vi "SPI MPU9250.vi"() -> ()   [LabVIEW 2020, in "CTI-Scratchpad.lvlib"]
uses:
  CTI-Scratchpad.lvlib
  CTI/SPI Config.ctl
  CTI/SPI Mode.ctl
  CTI/SPI Pins.ctl
  CTI/GPIO Number.ctl
  CTI/SPI Number.ctl
  CTI/GPIO Direction.ctl
  CTI/Session/Session.lvclass
  6879a345-385a-4bff-b9a2-dde094eab613.vi
  CTI/SPI/SPI.lvclass
  CTI/VisaComms/VisaComms.lvclass
  CTI/SPI CS/SPI CS.lvclass
  CTI/CTI.lvlib
panel:
  out "ID":string
  out "Chart":T1(graph)
  in  "stop":bool
  out "error out":errorcluster={"status"=FALSE, "code"=1073676294, "source"="VISA Read in CTI-Visa.lvlib:Read Response.vi->CTI-Visa.lvlib:Read SPI.vi->CTI-Visa-DeviceLib.lvlib:SPI Read Register.vi->CTI-Visa-Scratchpad.lvlib:SPI MPU9250.vi"}
  in  "CS GPIO":T2=5
  in  "Baud":u32=500000 format="%.0p"
  in  "SPI #":T3
  in  "SPI Config":T4={"Mode"=0, "Data Bits"=8, "Pins"={"TX GPIO"=7, "RX GPIO"=4, "SCK GPIO"=6}}
  in  "Port":refnum<visa-resource-name>="COM4"
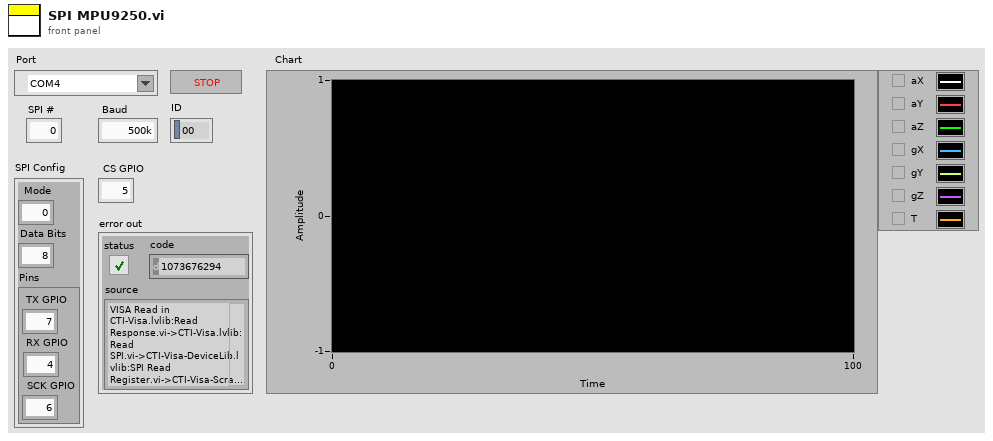
[diagram p1: front panel]
types:
  T1 = cluster{"X":u16, "Y":u16, "Z":u16, "X":u16, "Y":u16, "Z":u16, "T":u16}
  T2 = typedef "CTI.lvlib/GPIO Number.ctl" = i8
  T3 = typedef "CTI.lvlib/SPI Number.ctl" = i8
  T4 = typedef "CTI.lvlib/SPI Config.ctl" = cluster{"Mode":T5, "Data Bits":i8, "Pins":T6}
  T5 = typedef "CTI.lvlib/SPI Mode.ctl" = i8
  T6 = typedef "CTI.lvlib/SPI Pins.ctl" = cluster{"TX GPIO":T2, "RX GPIO":T2, "SCK GPIO":T2}
  T7 = typedef "CTI.lvlib/GPIO Direction.ctl" = enum16{"In", "Out"}
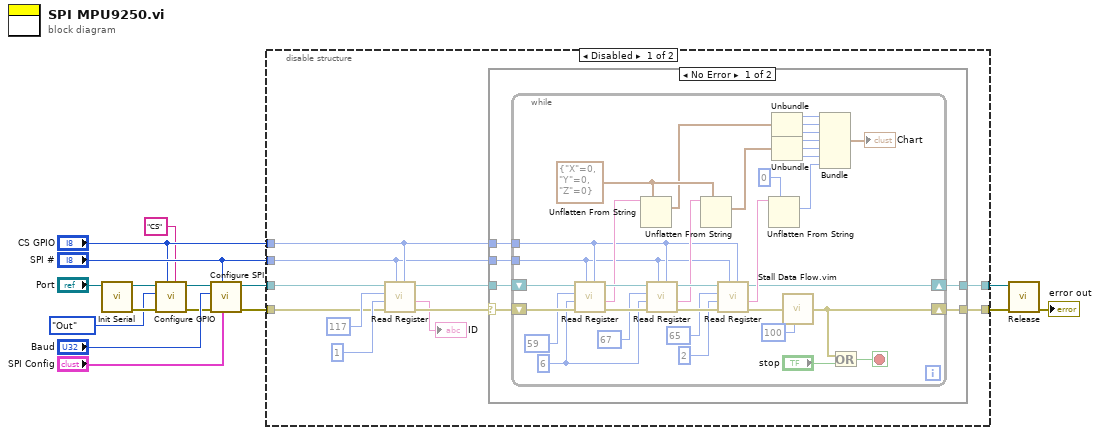
[diagram p0: block diagram]
diagram:
  n1 = call "Init Serial.vi"("VISA resource name in"="Port") -> ("error out"=w8:errorcluster, "Session"=w5:refnum<class "Session.lvclass">)  [unwired: 8 in, 1 out]
  n2 = call "Configure GPIO.vi"("Purpose (\"GPIO\")"="CS" ("Purpose (\"GPIO\")"), "GPIO #"="CS GPIO", "error in (no error)"=w8, "GPIO Direction"=GPIO_Direction."Out", "Session in"=w5) -> ("error out"=w6:errorcluster, "Session out"=w4:refnum<class "Session.lvclass">)  [unwired: 5 in]
  n3 = call "Configure SPI.vi"("SPI Config"="SPI Config", "SPI #"="SPI #", "error in (no error)"=w6, "Baud"="Baud", "Session in"=w4) -> ("error out"=w10:errorcluster, "Session out"=w11:refnum<class "Session.lvclass">)  [unwired: 5 in]
  n4 = disable-structure shown="Disabled" {
    disable-tunnel: [w27 _] -> w15
    disable-tunnel: [w26 _] -> w14
    disable-tunnel: w11 -> [w18 _]
    disable-tunnel: w10 -> [w17 _]
    disable-tunnel: "CS GPIO" -> [w20 _]
    disable-tunnel: "SPI #" -> [w19 _]
    frame Disabled {
      n5 = call "Read Register.vi"("CS (None)"=w20, "SPI"=w19, "error in (no error)"=w17, "Len"=u8 1, "Register"=u8 117, "Session In"=w18) -> ("error out"=w25:errorcluster, "Data"=→"ID":string, "Session Out"=w24:refnum<class "Session.lvclass">)  [unwired: 3 in]
      n6 = case shown="No Error" w25 {
        selector: w25 -> [w33 w68]
        tunnel: w24 -> [w32 w69]
        tunnel: [w31 w69] -> w27
        tunnel: [w30 w68] -> w26
        tunnel: w20 -> [w29 _]
        tunnel: w19 -> [w28 _]
        frame No Error {
          n7 = while {
            shift-right: [w58] -> w30
            shift-left: w33 -> [w67]
            shift-right: [w40] -> w31
            shift-left: w32 -> [w42]
            tunnel: w29 -> [w38]
            tunnel: w28 -> [w37]
            stop <- w59 stop-if-true
            w54 = cluster{"X":u16, "Y":u16, "Z":u16} {"X"=0, "Y"=0, "Z"=0}
            w63 = u8 6 ("Len")
            n8 = call "Read Register.vi"("CS (None)"=w38, "SPI"=w37, "error in (no error)"=w67, "Len"=w63, "Register"=u8 59, "Session In"=w42) -> ("error out"=w64:errorcluster, "Data"=w56:string, "Session Out"=w65:refnum<class "Session.lvclass">)  [unwired: 3 in]
            n9 = Unflatten From String(type=w54, binary string=w56) -> (value=w51:cluster{"X":u16, "Y":u16, "Z":u16})  [unwired: 3 in, 2 out]
            n10 = call "Read Register.vi"("CS (None)"=w38, "SPI"=w37, "error in (no error)"=w64, "Len"=w63, "Register"=u8 67, "Session In"=w65) -> ("error out"=w61:errorcluster, "Data"=w55:string, "Session Out"=w62:refnum<class "Session.lvclass">)  [unwired: 3 in]
            n11 = Unflatten From String(type=w54, binary string=w55) -> (value=w50:cluster{"X":u16, "Y":u16, "Z":u16})  [unwired: 3 in, 2 out]
            n12 = call "Read Register.vi"("CS (None)"=w38, "SPI"=w37, "error in (no error)"=w61, "Len"=u8 2, "Register"=u8 65, "Session In"=w62) -> ("error out"=w41:errorcluster, "Data"=w52:string, "Session Out"=w40:refnum<class "Session.lvclass">)  [unwired: 3 in]
            n13 = Unflatten From String(type=u16 0 ("T"), binary string=w52) -> (value=w43:u16)  [unwired: 3 in, 2 out]
            n14 = Unbundle(w51) -> ("X"=w49:u16, "Y"=w48:u16, "Z"=w47:u16)
            n15 = Unbundle(w50) -> ("X"=w46:u16, "Y"=w45:u16, "Z"=w44:u16)
            n16 = call "Stall Data Flow.vim"("value in"=w41, "milliseconds to wait"=u32 100) -> ("value out"=w58:errorcluster)  [unwired: 1 out]
            n17 = Bundle("X"=w49, "Y"=w48, "Z"=w47, "X"=w46, "Y"=w45, "Z"=w44, "T"=w43) -> (→"Chart":T1)  [unwired: 1 in]
            n18 = Or(x=w58, y="stop") -> (x .or. y?=w59:bool)
          }
        }
        frame Error {
        }
      }
    }
    frame Enabled {
    }
  }
  n19 = call-dynamic "Release.vi"("error in (no error)"=w14, "Session in"=w15) -> ("error out"=→"error out":errorcluster)  [unwired: 9 in]
